vi "Occurrence_LV2.vi"(0 "Without data DVR reference in":refnum<data-value>, 11 "Error In":errorcluster, 13 "Operation":enum16{"Init", "Read", "Write"}(ring)) -> (4 "Without data DVR reference out":refnum<data-value>, 15 "Error Out":errorcluster)   [LabVIEW 2020, in "Data Communication Transmitter.lvlib"]
doc: "This VI is used save the reference of the occurrence to get the occurrence in the receiver."
uses:
  Data Communication Transmitter.lvlib
  Classes/Children/Intra-Application/Children/Without data/Without Data.lvclass
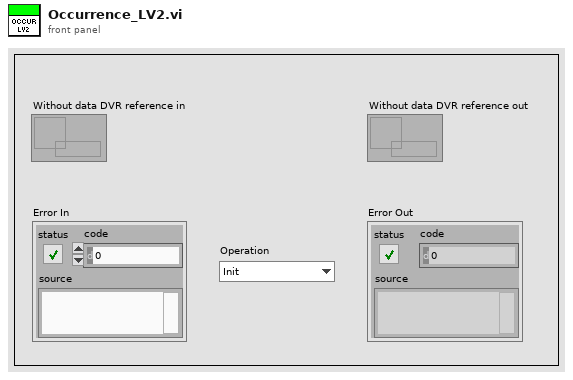
[diagram p1: front panel]
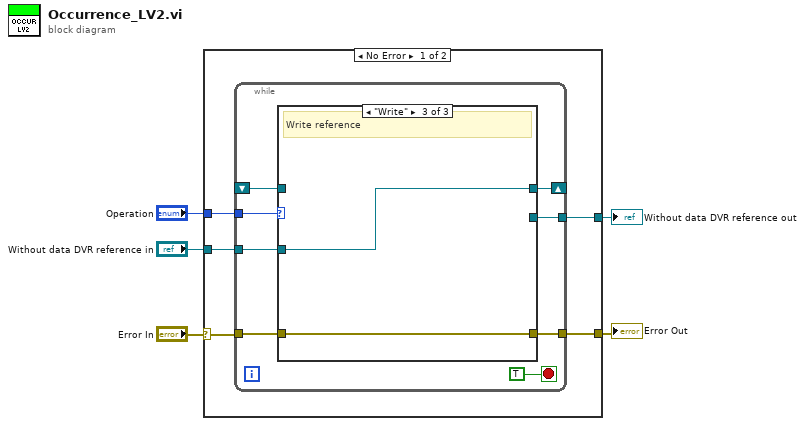
[diagram p0: block diagram]
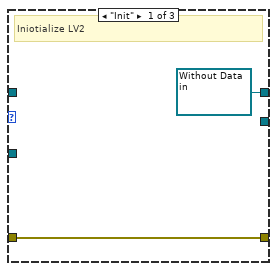
[diagram p2: hidden frame]
diagram:
  n1 = case shown="No Error" "Error In" {
    selector: "Error In" -> [w6 w25]
    tunnel: [w10 w25] -> w5
    tunnel: "Operation" -> [w9 _]
    tunnel: [w8 _] -> w1
    tunnel: "Without data DVR reference in" -> [w7 _]
    frame No Error {
      n2 = while {
        shift-right: [w14] -> _
        shift-left: _ -> [w15]
        tunnel: w6 -> [w18]
        tunnel: [w17] -> w10
        tunnel: w9 -> [w16]
        tunnel: [w13] -> w8
        tunnel: w7 -> [w12]
        stop <- TRUE stop-if-true
        n3 = case shown="\"Write\"" w16 {
          tunnel: [w20 w21 w24] -> w17
          tunnel: w18 -> [w20 w21 w24]
          tunnel: [refnum<data-value> refnum ("Without data DVR reference in") w22 w23] -> w14
          tunnel: w15 -> [_ w22 _]
          tunnel: [_ w22 _] -> w13
          tunnel: w12 -> [_ _ w23]
          frame "Init" {
            # "Iniotialize LV2"
          }
          frame "Read" {
            # "Read reference"
          }
          frame "Write" {
            # "Write reference"
          }
        }
      }
    }
    frame Error {
    }
  }
  "Error Out" <- w5
  "Without data DVR reference out" <- w1
